vi "HFRR ADV v11.vi"() -> ()   [LabVIEW 2025] (continued)
                  tunnel: [_ _ _ w5655 _ _ _] -> w5578
                  tunnel: w5568 -> [_ _ _ _ _ _ w5688]
                  tunnel: [_ _ _ _ _ _ w5687] -> w5564
                  tunnel: [_ _ _ _ _ w5667 _] -> w5563
                  tunnel: [_ _ _ _ w5660 _ _] -> w5562
                  frame #0 {
                    n4161 = local read "NORMAL LOAD"() -> (w5629:dbl)
                    n4162 = Number To Fractional String(number=w5629, width (-)=i16 10, precision (6)=i16 4) -> (F-format string=w5632:string)  [unwired: 1 in]
                    n4163 = Concatenate Strings("NormalLoad\":\"", w5632, w5630) -> (w5631:string)
                  }
                  frame #1 {
                    n4164 = local read "Temp"() -> (w5637:dbl)
                    n4165 = Number To Fractional String(number=w5637, width (-)=i16 10, precision (6)=i16 4) -> (F-format string=w5640:string)  [unwired: 1 in]
                    n4166 = Concatenate Strings("Temperature\":\"", w5640, w5638) -> (w5639:string)
                  }
                  frame #2 {
                    n4167 = local read "cof"() -> (w5643:dbl)
                    n4168 = Number To Fractional String(number=w5643, width (-)=i16 10, precision (6)=i16 4) -> (F-format string=w5647:string)  [unwired: 1 in]
                    n4169 = Concatenate Strings("FrictionalForce\":\"", w5647, w5645) -> (w5646:string)
                  }
                  frame #3 {
                    n4170 = local read "Set Hz"() -> (w5651:dbl)
                    n4171 = Multiply(x=w5651, y=60.0) -> (x*y=w5650:dbl)
                    n4172 = Number To Fractional String(number=w5650, width (-)=i16 10, precision (6)=i16 4) -> (F-format string=w5656:string)  [unwired: 1 in]
                    n4173 = Concatenate Strings("Speed\":\"", w5656, w5653) -> (w5655:string)
                  }
                  frame #4 {
                    n4174 = local read "Stroke Ln"() -> (w5659:dbl)
                    n4175 = Number To Fractional String(number=w5659, width (-)=i16 10, precision (6)=i16 4) -> (F-format string=w5663:string)  [unwired: 1 in]
                    n4176 = Concatenate Strings("LinearDeformation\":\"", w5663, w5661) -> (w5660:string)
                  }
                  frame #5 {
                    n4177 = local read "AIR TEMP"() -> (w5666:dbl)
                    n4178 = local read "Json St Flg"() -> (w5668:bool)
                    n4179 = local read "Json End Flg"() -> (w5669:bool)
                    n4180 = Number To Fractional String(number=w5666, width (-)=i16 10, precision (6)=i16 4) -> (F-format string=w5672:string)  [unwired: 1 in]
                    n4181 = Concatenate Strings("Vibration\":\"", w5672, w5670) -> (w5667:string)
                    n4182 = And(x=w5668, y=w5669) -> ()  [unwired: 1 out]
                  }
                  frame #6 {
                    n4183 = local read "Json End Flg"() -> (w5676:bool)
                    n4184 = Get Date/Time In Seconds() -> (seconds since 1Jan1904=w5684:timestamp)
                    n4185 = local read "Json St Flg"() -> (w5675:bool)
                    n4186 = To Double Precision Float(number=w5684) -> (double precision float=w5683:dbl)
                    n4187 = Subtract(x=w5683, y=2082844800.0) -> (x-y=w5681:dbl)
                    n4188 = Number To Fractional String(number=w5681, width (-)=i16 12, precision (6)=i16 0) -> (F-format string=w5678:string)  [unwired: 1 in]
                    n4189 = case shown="True" w5676 {
                      tunnel: ["" w5691] -> w5685
                      tunnel: w5678 -> [_ w5692]
                      tunnel: w5677 -> [_ w5690]
                      frame False {
                      }
                      frame True {
                        n4190 = local write "Json End Flg"(FALSE ("Json St Flg")) -> ()
                        n4191 = Concatenate Strings("End\": \"", w5692, w5690) -> (w5691:string)
                      }
                    }
                    n4192 = case shown="True" w5675 {
                      tunnel: [w5695 w5698] -> w5686
                      tunnel: w5678 -> [_ w5699]
                      tunnel: w5677 -> [_ w5696]
                      frame False {
                        n4193 = local read "St Str"() -> (w5695:string)
                      }
                      frame True {
                        n4194 = Concatenate Strings("Start\":\"", w5699, w5696) -> (w5698:string)
                        "St Str" <- w5698
                        n4195 = local write "Json St Flg"(FALSE ("Json St Flg")) -> ()
                      }
                    }
                    n4196 = Concatenate Strings(w5686, w5685, w5688) -> (w5687:string)
                  }
                }
                n4197 = local read "FILE"() -> (w5556:string)
                n4198 = Concatenate Strings("\",\"OperatorID\":\"" ("string"), "Operator ID") -> (w5559:string)
                n4199 = Concatenate Strings("\",\"DatasetTitle\":\"" ("string"), w5556) -> (w5558:string)
                n4200 = Concatenate Strings("\",\"SerialNumber\":\"" ("string"), "Serial No") -> (w5588:string)
                n4201 = Concatenate Strings("\",\"ModelNumber\":\"" ("string"), "Model No") -> (w5587:string)
                n4202 = Concatenate Strings(w5588, w5587) -> (w5570:string)
                n4203 = Concatenate Strings("{\"SecretKey\":\"", "Secret Key", w5570, w5559, w5558, "\",\"Samples\":[") -> (w5575:string)
                n4204 = Concatenate Strings(w5577, w5581, w5580, w5579, w5578, w5562, w5563, w5564) -> (w5576:string)
                n4205 = Concatenate Strings(w5575, w5576, "]}") -> (w5574:string)
                n4206 = stacked-sequence {
                  tunnel: w5574 -> [w5603 _ _]
                  tunnel: [_ _ w5620] -> _
                  frame #0 {
                    (unwired) FALSE ("convert eol (F)")
                    w5605 = enum16{"start", "end", "current"}."start" ("pos mode (0:2)")
                    n4207 = Path To String(path="Path") -> (string=w5611:string)
                    n4208 = Concatenate Strings(w5611, "\\", "Data File Name") -> (w5613:string)
                    n4209 = local write "standard output"(" ") -> ()
                    n4210 = String To Path(string=w5613) -> (path=w5602:path)
                    n4211 = call <vilib>:"Open_Create_Replace File.vi"("advisory dialog? (display:T)"=FALSE, "function (open:0)"=T28."create or replace", "file path"=w5602) -> ("error out"=w5616:errorcluster, "refnum"=w5615:refnum<file>)  [unwired: 5 in, 2 out]
                    n4212 = Set File Position(refnum=w5615, from (0:start)=w5605, error in=w5616) -> (refnum out=w5596:refnum<file>, error out=w5595:errorcluster)  [unwired: 1 in]
                    n4213 = Write to Binary File(file (use dialog)=w5596, data=" ", error in=w5595, 5:FALSE ("prepend array or string size? (T)")) -> (refnum out=w5606:refnum<file>, error out=w5607:errorcluster)  [unwired: 2 in, 1 out]
                    n4214 = Set File Position(offset (in bytes) (0)=w5605, refnum=w5606, error in=w5607) -> (refnum out=w5599:refnum<file>, error out=w5598:errorcluster)  [unwired: 1 in]
                    n4215 = Write to Binary File(file (use dialog)=w5599, data=w5603, error in=w5598, 5:FALSE ("prepend array or string size? (T)")) -> (error out=w5601:errorcluster)  [unwired: 2 in, 2 out]
                    n4216 = flat-sequence {
                      tunnel: w5602 -> [w5618]
                      tunnel: w5601 -> [_]
                      frame #0 {
                        n4217 = call <vilib>:"Read Characters From File.vi"("file path (dialog if empty)"=w5618) -> ("character string"=→"JSON string":string)  [unwired: 5 in, 3 out]
                      }
                    }
                    "SinglePoint" <- w5603
                  }
                  frame #1 {
                  }
                  frame #2 {
                    (unwired) "\"Stored\": true" ("string")
                    n4218 = call <vilib>:"System Exec.vi"("run minimized? (F)"=TRUE, "wait until completion? (T)"=TRUE, "working directory"=path "C:/LAB-IQ-NXT", "command line"="C:\\LAB-IQ-NXT\\JPost.bat") -> ("standard error"=→"Respose From Server":string, "standard output"=w5623:string)  [unwired: 4 in, 2 out]
                    "standard output" <- w5623
                    n4219 = Match Pattern(string=w5623, regular expression="JSON Check String") -> (match substring=w5621:string, offset past match=w5620:i32)  [unwired: 1 in, 2 out]
                    n4220 = Equal?(x=w5621, y="JSON Check String") -> (x = y?=→"Upload \nConfirmed":bool)
                  }
                }
              }
            }
            n4221 = local read "Quit"() -> (w5544:bool)
          }
        }
      }
    }
    frame Enabled {
    }
  }
  n4222 = disable-structure shown="Disabled" {
    disable-tunnel: _ -> [w5706 _]
    frame Disabled {
      n4223 = while {
        shift-right: [w5714] -> w5702
        shift-left: _ -> [w5715]
        shift-right: [w5712] -> w5703
        shift-left: errorcluster {"status"=TRUE, "code"=0, "source"="Init"} ("error out") -> [w5713]
        shift-right: [w5710] -> _
        shift-left: "" -> [w5711]
        tunnel: [w5708] -> _
        tunnel: w5706 -> [_]
        i -> [w5708]
        stop <- w5707 stop-if-true
        n4224 = flat-sequence {
          tunnel: [w5716] -> w5709
          frame #0 {
            n4225 = Wait (ms)(milliseconds to wait=10.0 ("Delay")) -> (millisecond timer value=w5716:u32)
          }
        }
        n4226 = case shown="No Error" w5713 {
          selector: w5713 -> [w5749 w5871]
          tunnel: [w5731 w5873] -> w5714
          tunnel: [w5730 w5872] -> w5712
          tunnel: w5715 -> [w5750 w5865]
          tunnel: w5711 -> [w5729 w5864]
          tunnel: [w5728 w5864] -> w5710
          tunnel: w5709 -> [_ _]
          frame No Error {
            n4227 = Concatenate Strings("COMMAND", "\r", "\n") -> (w5740:string)
            n4228 = case shown="True" "Measure" {
              tunnel: w5750 -> [w5776 w5783]
              tunnel: w5749 -> [w5775 w5782]
              tunnel: [w5776 w5781] -> w5748
              tunnel: [w5775 w5780] -> w5727
              tunnel: w5740 -> [_ w5779]
              frame False {
              }
              frame True {
                n4229 = VISA Write(VISA resource name=w5783, write buffer=w5779, error in (no error)=w5782) -> (VISA resource name out=w5781:refnum<visa-resource-name>, error out=w5780:errorcluster)  [unwired: 1 out]
                n4230 = local write "Read String"("") -> ()
                n4231 = local write "Measure"(FALSE) -> ()
              }
            }
            n4232 = property class="Instr"(reference=w5748, error in=w5727) -> (reference out=w5747:refnum<visa-resource-name>, error out=w5746:errorcluster, "Serial Settings:Number of Bytes at Serial Port"=w5745:u32)
            n4233 = Greater?(x=w5745, y=u32 100) -> (0:w5743:bool)
            n4234 = case shown="True" w5743 {
              tunnel: w5747 -> [w5786 w5811]
              tunnel: w5746 -> [w5785 w5810]
              tunnel: w5745 -> [_ w5809]
              tunnel: [w5786 w5808] -> w5733
              tunnel: [w5785 w5807] -> w5732
              tunnel: w5729 -> [w5784 w5806]
              tunnel: [w5784 ""] -> w5728
              frame False {
              }
              frame True {
                w5796 = u32 6 ("y")
                # "Page 84 of \nmanual"
                n4235 = VISA Read(VISA resource name=w5811, byte count=w5809, error in (no error)=w5810) -> (VISA resource name out=w5808:refnum<visa-resource-name>, read buffer=w5804:string, error out=w5807:errorcluster)  [unwired: 1 out]
                n4236 = while {
                  tunnel: w5804 -> [w5860]
                  tunnel: [w5856] -> w5798 mode=indexing
                  tunnel: [w5850] -> w5802 mode=indexing
                  tunnel: [w5848] -> _
                  i -> [w5848]
                  stop <- w5853 stop-if-true
                  n4237 = String Subset(string=w5860, offset (0)=w5848) -> (substring=w5855:string)  [unwired: 1 in]
                  n4238 = String To Byte Array(string=w5855) -> (unsigned byte array=w5859:u8[])
                  n4239 = String Length(string=w5855) -> (length=w5854:i32)
                  n4240 = Index Array(array=w5859) -> (element=w5858:u8)  [unwired: 1 in]
                  n4241 = Equal To 0?(x=w5854) -> (x = 0?=w5853:bool)
                  n4242 = Number To Boolean Array(number=w5858) -> (Boolean array=w5852:bool[])
                  n4243 = Reverse 1D Array(array=w5852) -> (reversed array=w5851:bool[])
                  n4244 = And(x=w5852, y=bool[] [FALSE, FALSE, FALSE, FALSE, FALSE, FALSE, TRUE, TRUE] ("Boolean array")) -> (x .and. y?=w5856:bool[])
                  n4245 = And(x=w5851, y=bool[] [FALSE, FALSE, TRUE, TRUE, TRUE, TRUE, TRUE, TRUE] ("Boolean array")) -> (x .and. y?=w5850:bool[])
                }
                n4246 = Concatenate Strings(w5806, w5804) -> (→"Read String":string)
                n4247 = while {
                  tunnel: w5798 -> [w5847] mode=indexing
                  tunnel: [w5843] -> w5801
                  i -> [w5843]
                  stop <- w5844 stop-if-true
                  n4248 = Search 1D Array(1D array=w5847, element=TRUE) -> (index of element=w5845:i32)  [unwired: 1 in]
                  n4249 = Less Than 0?(x=w5845) -> (x < 0?=w5844:bool)
                }
                n4250 = Delete From Array(array=w5802, length=w5801, index (row)=0) -> (array with subset deleted=w5797:bool[][])  [unwired: 1 in, 1 out]
                n4251 = Array Size(array=w5797) -> (size(s)=w5799:i32[])
                n4252 = Index Array(array=w5799) -> (element=w5791:i32)  [unwired: 1 in]
                n4253 = Greater?(x=w5791, y=w5796) -> (0:w5794:bool)
                n4254 = Subtract(x=w5791, y=w5796) -> (x-y=w5795:u32)
                n4255 = Select(t=w5795, s=w5794, f=u32 0) -> (s? t:f=w5792:u32)
                n4256 = while {
                  tunnel: w5797 -> [w5830]
                  tunnel: [w5832] -> w5790 mode=indexing
                  tunnel: w5792 -> [w5814]
                  i -> [w5831]
                  stop <- w5829 stop-if-true
                  w5821 = 6 ("index")
                  w5820 = 2 ("length")
                  # "Page 65 of \nmanual"
                  n4257 = Multiply(x=u32 3 ("y"), y=w5831) -> (x*y=w5828:u32)
                  n4258 = Divide(x=u32 102 ("y"), y=u32 65520) -> (x/y=w5838:dbl)
                  n4259 = Greater Or Equal?(x=w5828, y=w5814) -> (x >= y?=w5829:bool)
                  n4260 = Index Array(array=w5830, index (row) #1=w5828) -> (element #1=w5826:bool[], element #2=w5825:bool[], element #3=w5824:bool[])  [unwired: 5 in]
                  n4261 = Reverse 1D Array(array=w5826) -> (reversed array=w5819:bool[])
                  n4262 = Reverse 1D Array(array=w5825) -> (reversed array=w5823:bool[])
                  n4263 = Reverse 1D Array(array=w5824) -> (reversed array=w5822:bool[])
                  n4264 = Delete From Array(array=w5819, length=w5820, index=w5821) -> (array with subset deleted=w5815:bool[])  [unwired: 1 out]
                  n4265 = Delete From Array(array=w5823, length=w5820, index=w5821) -> (array with subset deleted=w5816:bool[])  [unwired: 1 out]
                  n4266 = Delete From Array(array=w5822, length=w5820, index=w5821) -> (array with subset deleted=w5817:bool[])  [unwired: 1 out]
                  n4267 = Insert Into Array(array=bool[] [] ("Boolean array"), new element #1=w5815, new element #2=w5816, new element #3=w5817) -> (w5818:bool[])  [unwired: 1 in]
                  n4268 = Boolean Array To Number(Boolean array=w5818) -> (number=w5827:u32)
                  n4269 = Multiply(x=w5838, y=w5827) -> (x*y=w5837:dbl)
                  n4270 = Decrement(x=w5837) -> (x-1=w5836:dbl)
                  n4271 = Divide(x=w5836, y=u32 100) -> (x/y=w5834:dbl)
                  n4272 = Multiply(x=w5834, y=u32 10) -> (x*y=w5832:dbl)
                }
                n4273 = Delete From Array(array=w5790) -> (array with subset deleted=w5789:dbl[])  [unwired: 2 in, 1 out]
                "Waveform Graph 5" <- w5789
                "Waveform Chart 3" <- w5789
                n4274 = call-poly <vilib>:"Mean.vi"("X"=w5789) -> ("mean"=w5788:dbl)  [unwired: 1 out]
                "Measure_LDS" <- w5788
                n4275 = case shown="True" "Zero 4" {
                  tunnel: w5788 -> [_ w5813]
                  frame False {
                  }
                  frame True {
                    n4276 = local write "Zero 4"(FALSE ("Zero 4")) -> ()
                    "z_measure" <- w5813
                  }
                }
              }
            }
            n4277 = local read "Measure_LDS"() -> (w5723:dbl)
            n4278 = local read "Disp (mm)"() -> (w5722:dbl)
            n4279 = local read "Boolean 7"() -> (w5721:bool)
            n4280 = local read "Boolean 8"() -> (w5720:bool)
            n4281 = case shown="True" "Boolean 8" {
              tunnel: w5722 -> [_ w5753]
              tunnel: w5723 -> [_ w5752]
              frame False {
              }
              frame True {
                n4282 = local read "Captured Values 2"() -> (w5756:dbl[][])
                n4283 = Build Array(w5753, w5752) -> (w5751:dbl[])
                n4284 = Build Array (concatenate)(w5756, w5751) -> (w5754:dbl[][])
                n4285 = local write "Captured Values 2"(w5754) -> ()
                n4286 = local write "Boolean 8"(FALSE ("Boolean 8")) -> ()
              }
            }
            n4287 = call "Build XY Graph"("Enable"=w5720, "Reset"=w5721, "Y Input"=w5723, "X Input"=w5722) -> ("XY Graph"=→"?":cluster{"Y":dbl[], "Y":dbl[]}[])  [unwired: 6 in, 1 out]
            n4288 = case shown="True" "Boolean 9" {
              frame False {
              }
              frame True {
                n4289 = local read "Captured Values 2"() -> (w5758:dbl[][])
                n4290 = Index Array(array=w5758, index (col) #1=0 ("disabled index (col)"), index (col) #2=1 ("index (col)")) -> (element #1=w5761:dbl[], element #2=w5760:dbl[])  [unwired: 2 in]
                n4291 = call <vilib>:"Linear Fit.vi"("Y"=w5761, "X"=w5760) -> ("slope"=→"Slope":dbl, "intercept"=→"Intercept":dbl)  [unwired: 9 in, 3 out]
                n4292 = local write "Boolean 9"(FALSE ("Boolean 9")) -> ()
              }
            }
            n4293 = case shown="True" "Boolean 7" {
              frame False {
              }
              frame True {
                n4294 = local write "Captured Values 2"(dbl[][] [] ("Captured Values")) -> ()
                n4295 = local write "Boolean 7"(FALSE ("Boolean 7")) -> ()
              }
            }
            n4296 = Concatenate Strings("COMMAND 2", "\r", "\n") -> (w5735:string)
            n4297 = case shown="True" "Measure 2" {
              tunnel: w5733 -> [w5768 w5774]
              tunnel: w5732 -> [w5767 w5773]
              tunnel: [w5768 w5772] -> w5731
              tunnel: [w5767 w5771] -> w5730
              tunnel: w5735 -> [_ w5770]
              frame False {
              }
              frame True {
                n4298 = local write "Measure 2"(FALSE ("WRITE")) -> ()
                n4299 = VISA Write(VISA resource name=w5774, write buffer=w5770, error in (no error)=w5773) -> (VISA resource name out=w5772:refnum<visa-resource-name>, error out=w5771:errorcluster)  [unwired: 1 out]
              }
            }
          }
          frame Error {
            w5863 = u16 10 items=["1.0"=10, "1.5"=15, "2.0"=20] ("stop bits (10: 1 bit)")
            n4300 = Wait (ms)(milliseconds to wait=u32 20) -> ()  [unwired: 1 out]
            n4301 = VISA Close(VISA resource name=w5865, error in (no error)=w5871) -> (error out=w5870:errorcluster)
            n4302 = call <vilib>:"Clear Errors.vi"("error in (no error)"=w5870) -> ("error out"=w5869:errorcluster)  [unwired: 5 in, 1 out]
            n4303 = call-poly "VISA Configure Serial Port"("VISA resource name"="Laser Disp Sensor", "timeout (10sec)"=u32 200, "Enable Termination\nChar (T)"=TRUE ("Enable Termination\nChar (T)"), "baud rate (9600)"=u32 921600, "error in (no error)"=w5869, "stop bits (10: 1 bit)"=w5863) -> ("VISA resource name out"=w5873:refnum<visa-resource-name>, "error out"=w5872:errorcluster)  [unwired: 8 in]
          }
        }
        n4304 = local read "Quit"() -> (w5707:bool)
      }
      n4305 = VISA Close(VISA resource name=w5702, error in (no error)=w5703) -> (error out=w5701:errorcluster)
      n4306 = call <vilib>:"Clear Errors.vi"("error in (no error)"=w5701) -> ()  [unwired: 5 in, 2 out]
    }
    frame Enabled {
    }
  }
  n4307 = disable-structure shown="Disabled" {
    disable-tunnel: _ -> [w5878 _]
    frame Disabled {
      n4308 = while {
        tunnel: [w5885] -> _
        shift-right: [w5882] -> w5875
        shift-left: _ -> [w5884]
        shift-right: [w5883] -> w5876
        shift-left: errorcluster {"status"=TRUE, "code"=0, "source"="Init"} ("error out") -> [w5881]
        tunnel: w5878 -> [_]
        i -> [w5885]
        stop <- w5879 stop-if-true
        n4309 = flat-sequence {
          tunnel: w5881 -> [w5976]
          tunnel: [w5976] -> w5880
          frame #0 {
            n4310 = Wait (ms)(milliseconds to wait=u32 50) -> ()  [unwired: 1 out]
          }
        }
        n4311 = case shown="No Error" w5880 {
          selector: w5880 -> [w5926 w5969]
          tunnel: w5884 -> [w5925 w5968]
          tunnel: [w5892 w5959] -> w5883
          tunnel: [w5893 w5967] -> w5882
          frame No Error {
            w5919 = T29 {"Mode"=enum."RTU", "Slave Address"=1} ("Serial Parameters")
            n4312 = call-poly <vilib>:"MB Serial Master Query (poly).vi"("VISA resource name"=w5925, "Starting Address"=i16 1000, "Quantity"=u16 1, "Timeout"=u32 1000, "error in"=w5926, "Serial Parameters"=w5919) -> ("VISA resource name out"=w5920:refnum<visa-resource-name>, "Input Registers"=w5922:u16[], "error out"=w5918:errorcluster)  [unwired: 10 in, 1 out]
            n4313 = Random Number (0-1)() -> (number: 0 to 1=w5907:dbl)
            n4314 = Index Array(array=w5922, index=0) -> (element=w5917:u16)
            n4315 = Subtract(x=w5907, y=0.5) -> (x-y=w5906:dbl)
            n4316 = Divide(x=w5917, y=10 ("index")) -> (x/y=w5911:dbl)
            n4317 = Multiply(x=w5906, y=0.5) -> (x*y=w5905:dbl)
            n4318 = Add(x=w5911, y=w5905) -> (x+y=w5910:dbl)
            n4319 = local read "Amb temp"() -> (w5894:dbl)
            n4320 = Multiply(x=w5910, y=0.2) -> (x*y=w5914:dbl)
            n4321 = Multiply(x=w5894, y=0.8) -> (x*y=w5912:dbl)
            n4322 = Add(x=w5914, y=w5912) -> (x+y=w5895:dbl)
            n4323 = local read "set temp old"() -> (w5889:dbl)
            n4324 = local write "Amb temp"(w5895) -> ()
            n4325 = Select(t="SetTemp 2", s="Heater", f=100.0) -> (s? t:f=w5890:dbl)
            n4326 = Not Equal?(x=w5890, y=w5889) -> (x != y?=w5888:bool)
            n4327 = case shown="True" w5888 {
              tunnel: w5920 -> [w5954 w5956]
              tunnel: [w5953 w5956] -> w5900
              tunnel: w5918 -> [w5952 w5955]
              tunnel: [w5951 w5955] -> w5898
              tunnel: w5890 -> [w5946 _]
              tunnel: w5919 -> [w5948 w5957]
              tunnel: [w5948 w5957] -> w5901
              frame True {
                n4328 = Multiply(x=w5946, y=10 ("index")) -> (x*y=w5945:dbl)
                n4329 = call-poly <vilib>:"MB Serial Master Query (poly).vi"("VISA resource name"=w5954, "Address"=u16 0, "Holding Register"=w5945, "Timeout"=u32 1000, "error in"=w5952, "Serial Parameters"=w5948) -> ("VISA resource name out"=w5953:refnum<visa-resource-name>, "error out"=w5951:errorcluster)  [unwired: 11 in, 1 out]
                "set temp old" <- w5946
              }
              frame False {
              }
            }
            n4330 = flat-sequence {
              tunnel: [w5927] -> _
              tunnel: [w5927] -> w5897
              tunnel: w5898 -> [w5927]
              frame #0 {
                n4331 = Wait (ms)(milliseconds to wait=u32 100) -> ()  [unwired: 1 out]
              }
            }
            n4332 = call "Elapsed Time12"("Time Target (s)"=2.0, "Auto Reset"=TRUE) -> ("Time has Elapsed"=w5902:bool)  [unwired: 10 in, 7 out]
            n4333 = case shown="True" w5902 {
              tunnel: w5901 -> [w5931 w5944]
              tunnel: [w5931 w5944] -> _
              tunnel: [w5930 w5942] -> w5893
              tunnel: w5900 -> [w5930 w5943]
              tunnel: [w5929 w5940] -> w5892
              tunnel: w5897 -> [w5929 w5941]
              frame False {
              }
              frame True {
                n4334 = call-poly <vilib>:"MB Serial Master Query (poly).vi"("VISA resource name"=w5943, "Starting Address"=i16 1003 ("Addr"), "Quantity"=u16 1, "Timeout"=u32 1000, "error in"=w5941, "Serial Parameters"=w5944) -> ("VISA resource name out"=w5942:refnum<visa-resource-name>, "Input Registers"=w5937:u16[], "error out"=w5940:errorcluster)  [unwired: 10 in, 1 out]
                n4335 = Index Array(array=w5937, index=0) -> (element=w5936:u16)
                n4336 = Divide(x=w5936, y=u16 10) -> (x/y=w5932:dbl)
                n4337 = local write "set temp old"(w5932) -> ()
                n4338 = local write "SetTemp"(w5932) -> ()
              }
            }
            "Error Code" <- w5892
            n4339 = Unbundle(w5892) -> ("status"=→"TK4 status":bool)  [unwired: 2 out]
            "SetTemp" <- "SetTemp 2"
          }
          frame Error {
            w5971 = u16 0 items=["None", "Odd", "Even", "Mark", "Space"] ("Parity")
            w5972 = u16 0 items=["None", "XON/XOFF", "RTS/CTS", "XON/XOFF & RTS/CTS", "DTR/DSR", "XON/XOFF & DTR/DSR"] ("Flow Control")
            n4340 = VISA Clear(VISA resource name=w5968, error in (no error)=w5969) -> (VISA resource name out=w5962:refnum<visa-resource-name>, error out=w5960:errorcluster)
            n4341 = VISA Close(VISA resource name=w5962, error in (no error)=w5960) -> (error out=w5961:errorcluster)
            n4342 = call <vilib>:"Clear Errors.vi"("error in (no error)"=w5961) -> ("error out"=w5970:errorcluster)  [unwired: 5 in, 1 out]
            n4343 = Unbundle By Name(T29 {"Mode"=enum."RTU", "Slave Address"=1} ("input cluster")) -> ("Mode"=w5973:enum16{"RTU", "ASCII"})
            n4344 = call <vilib>:"MB Serial Init.vi"("Timeout"=u32 100, "Flow Control"=w5972, "Mode"=w5973, "error in (no error)"=w5970, "Parity"=w5971, "Baud Rate"=u32 9600, "VISA resource name"="Lubrication System COM Port :") -> ("error out"=w5959:errorcluster, "VISA resource name out"=w5967:refnum<visa-resource-name>)  [unwired: 3 in]
            n4345 = local write "set temp old"(0.0 ("set temp old")) -> ()
            n4346 = Unbundle(w5959) -> ("status"=w5958:bool)  [unwired: 2 out]
            n4347 = case shown="True" w5958 {
              selector: w5958 -> [_ w5975]
              frame False {
              }
              frame True {
                n4348 = local write "TK4 status"(w5975) -> ()
              }
            }
          }
        }
        n4349 = local read "Quit"() -> (w5879:bool)
      }
      n4350 = VISA Close(VISA resource name=w5875, error in (no error)=w5876) -> (error out=w5874:errorcluster)
      n4351 = call <vilib>:"Clear Errors.vi"("error in (no error)"=w5874) -> ()  [unwired: 5 in, 2 out]
    }
    frame Enabled {
    }
  }
  "file count" <- 0 ("file count")
